vi "Configure Function.vi"(7 "FUNC":T1(ring), 8 "error in (no error)":errorcluster, 11 "VISA resource name":refnum<visa-resource-name>) -> (0 "error out":errorcluster, 3 "VISA resource name out":refnum<visa-resource-name>)   [LabVIEW 2018, in "Fluke 9500B.lvlib"]
uses:
  <instrlib>/Fluke 9500B/Fluke 9500B.lvlib
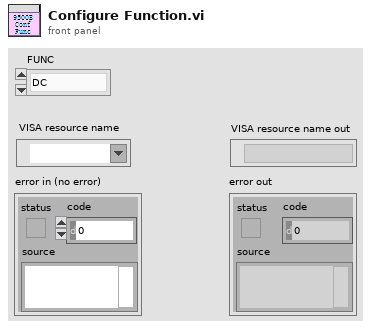
[diagram p1: front panel]
types:
  T1 = enum16{"DC", "SQU", "EDGE", "MARK", "SIN", "OPUL"}
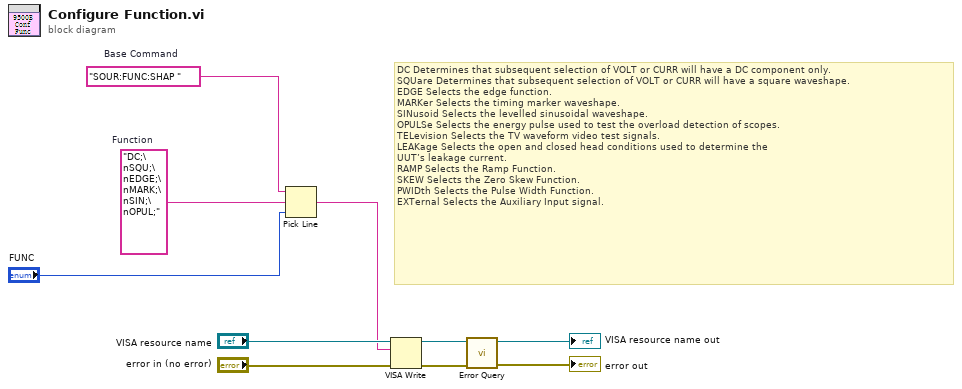
[diagram p0: block diagram]
diagram:
  w6 = "DC;\nSQU;\nEDGE;\nMARK;\nSIN;\nOPUL;"  # Function
  w7 = "SOUR:FUNC:SHAP "  # Base Command
  # "DC Determines that subsequent selection of VOLT or CURR will have a DC component only. \nSQUare Determines that subsequent selection of VOLT or CURR will have a square waveshape. \nEDGE Selects the edge function. \nMARKer Selects the timing marker waveshape. \nSINusoid Selects the levelled sinusoidal waveshape. \nOPULSe Selects the energy pulse used to test the overload detection of scopes. \nTELevision Selects the TV waveform video test signals. \nLEAKage Selects the open and closed head conditions used to determine the \nUUT’s leakage current. \nRAMP Selects the Ramp Function. \nSKEW Selects the Zero Skew Function. \nPWIDth Selects the Pulse Width Function. \nEXTernal Selects the Auxiliary Input signal."
  n1 = Pick Line(string ("")=w7, multi-line string=w6, line index="FUNC") -> (output string=w8:string)
  n2 = VISA Write(VISA resource name="VISA resource name", write buffer=w8, error in (no error)="error in (no error)") -> (VISA resource name out=w1:refnum<visa-resource-name>, error out=w2:errorcluster)  [unwired: 1 out]
  n3 = call <instrlib>:"Error Query.vi"("error in (no error)"=w2, "VISA resource name"=w1) -> ("error out"=→"error out":errorcluster, "VISA resource name out"=→"VISA resource name out":refnum<visa-resource-name>)  [unwired: 6 in, 2 out]
